vi "Do Request.vi"(7 "Processing In":refnum<class "Processing.lvclass">, 11 "CurrentStateController in":refnum<class "CurrentStateController.lvclass">) -> (0 "error out":errorcluster, 5 "Processing":refnum<class "Processing.lvclass">)   [LabVIEW 2022 SP3, in "VideoMux.lvlib" / "CurrentStateController.lvclass"]
uses:
  CurrentStateController.lvclass
  <vilib>/IlluminatedG/IG HTTP Server/HTTP Server/Processing/Processing.lvclass
  MuxAPI/MuxAPI.lvclass
  C:/Program Files (x86)/National Instruments/LabVIEW 2022/vi.lib/IlluminatedG/IG HTTP Server/HTTP Server/Service/Service.lvclass
  <vilib>/IlluminatedG/IG HTTP Server/HTTP Server/Processing/Processing.lvclass/Processing.ctl
  CurrentStateController.lvclass/CurrentStateController.ctl
  <vilib>/IlluminatedG/IG HTTP Utils/HTTP Utils/Response/Response.lvclass
  C:/dev/illuminatedg/TouchControl/VideoMux/MuxAPI/MuxAPI.lvclass
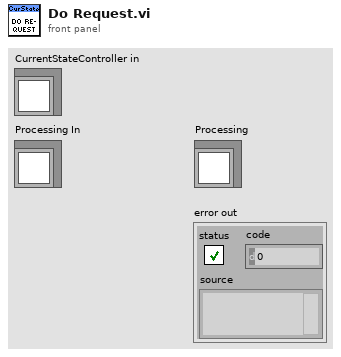
[diagram p1: front panel]
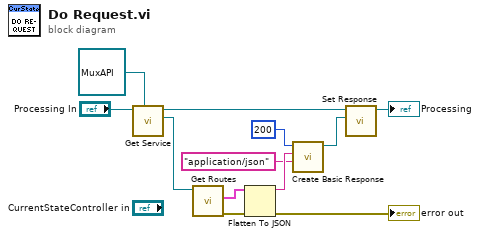
[diagram p0: block diagram]
diagram:
  n1 = call <vilib>:"Get Service.vi"("Service Type"=refnum<class "MuxAPI.lvclass"> refnum ("VideoMux.lvlib:MuxAPI.lvclass"), "Processing in"="Processing In") -> ("Service"=w11:refnum<class "MuxAPI.lvclass">, "Processing out"=w9:refnum<class "Processing.lvclass">)  [unwired: 7 in, 1 out]
  n2 = call "Get Routes.vi"("MuxAPI in"=w11) -> ("error out"=w3:errorcluster, "Routes"=w4:cluster{"Mux Route":i32[]}[])  [unwired: 8 in, 1 out]
  n3 = Flatten To JSON(anything=w4, error in (no error)=w3) -> (JSON string=w2:string, 11:→"error out":errorcluster)  [unwired: 1 in]
  n4 = call <vilib>:"Create Basic Response.vi"("Content-Type (text/plain)"="application/json" ("Payload"), "Payload"=w2, "Status Code"=u16 200) -> ("Response out"=w8:refnum<class "Response.lvclass">)  [unwired: 7 in, 1 out]
  n5 = call <vilib>:"Set Response.vi"("Response"=w8, "Processing in"=w9) -> ("Processing out"=→"Processing":refnum<class "Processing.lvclass">)  [unwired: 9 in]
